vi "test Connect at Local Address.vi"(8 "error in (no error)":errorcluster, 11 "TestCase in":refnum<class "Test TCP Stream Listener Connect.lvclass">) -> (0 "error out":errorcluster, 3 "TestCase out":refnum<class "Test TCP Stream Listener Connect.lvclass">)   [LabVIEW 2020, in "Test TCP Stream Listener Connect.lvclass"]
uses:
  Test TCP Stream Listener Connect.lvclass
  <vilib>/addons/_JKI Toolkits/VI Tester/TestCase.llb/TestCase.lvclass
  Source/Protocols/TCP Strategy/TCP Stream Listener/TCP Stream Listener.lvclass
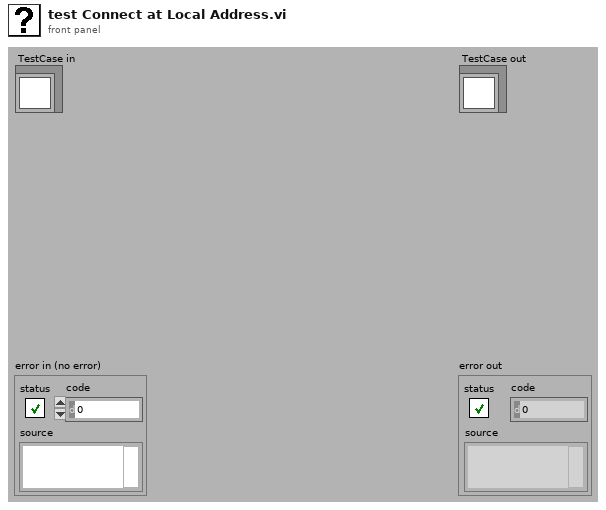
[diagram p1: front panel]
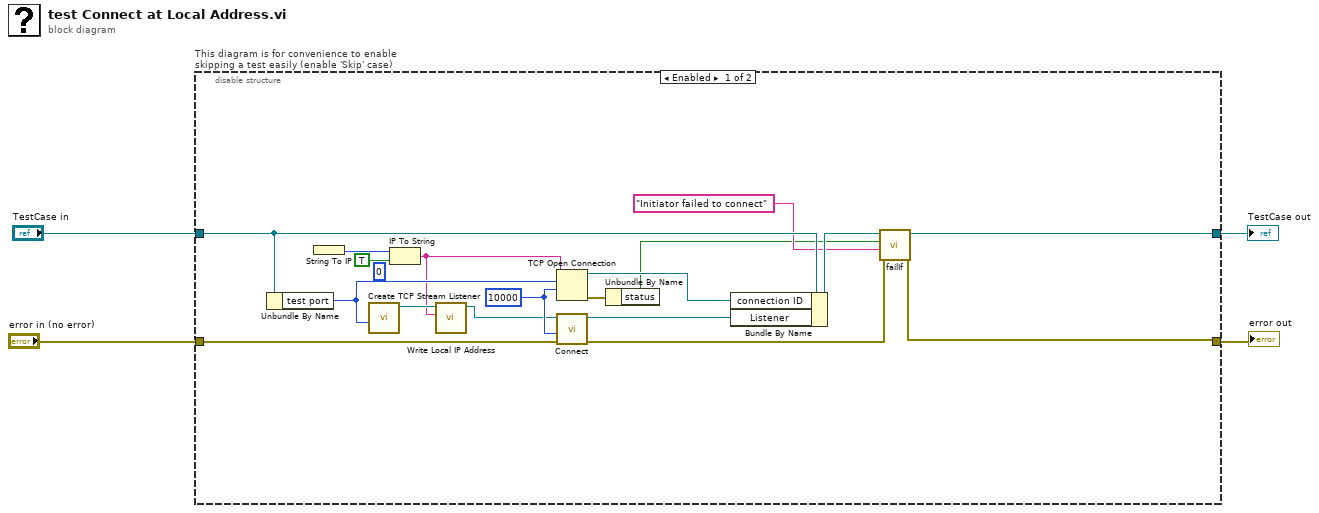
[diagram p0: block diagram]
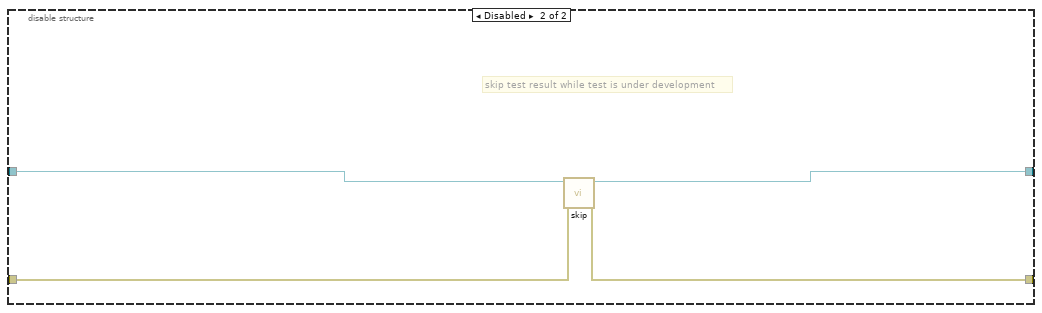
[diagram p2: hidden frame]
diagram:
  n1 = disable-structure "This diagram is for convenience to enable skipping a test easily (enable 'Skip' case)" shown="Enabled" {
    disable-tunnel: "TestCase in" -> [w18 w26]
    disable-tunnel: [w22 w24] -> w1
    disable-tunnel: [w21 w25] -> w3
    disable-tunnel: "error in (no error)" -> [w20 w23]
    frame Enabled {
      (unwired) u32 0 ("net address")
      w13 = 10000 ("timeout")
      n2 = Unbundle By Name(w18) -> ("test port"=w8:u16)
      n3 = String To IP() -> (0:w14:u32)  [unwired: 1 in]
      n4 = call "Create TCP Stream Listener.vi"("Local Port"=w8) -> ("TCP Stream Listener"=w7:refnum<class "TCP Stream Listener.lvclass">)  [unwired: 10 in]
      n5 = IP To String(1:TRUE ("dot notation? (F)"), 2:w14) -> (0:w5:string)
      n6 = call-dynamic "Write Local IP Address.vi"("Local IP"=w5, "TCP Stream Listener in"=w7) -> ("TCP Stream Listener out"=w6:refnum<class "TCP Stream Listener.lvclass">)  [unwired: 9 in]
      n7 = TCP Open Connection(address=w5, remote port or service name=w8, timeout ms (60000)=w13) -> (connection ID=w11:refnum<k5>, error out=w12:errorcluster)  [unwired: 2 in]
      n8 = call-dynamic "Connect.vi"("error in (no error)"=w20, "timeout"=w13, "TCP Stream Listener in"=w6) -> ("error out"=w19:errorcluster, "TCP Stream Listener out"=w9:refnum<class "TCP Stream Listener.lvclass">)  [unwired: 7 in]
      n9 = Unbundle By Name(w12) -> ("status"=w10:bool)
      n10 = Bundle By Name(cluster=w18, "connection ID"=w11, "Listener"=w9) -> (w17:refnum<class "Test TCP Stream Listener Connect.lvclass">)
      n11 = call-dynamic "failIf.vi"("error in (no error)"=w19, "message (\"\")"="Initiator failed to connect" ("message (\"\")"), "fail"=w10, "TestCase in"=w17) -> ("error out"=w21:errorcluster, "TestCase out"=w22:refnum<class "Test TCP Stream Listener Connect.lvclass">)  [unwired: 6 in]
    }
    frame Disabled {
      # "skip test result while test is under development"
      n12 = call <vilib>:"skip.vi"("error in (no error)"=w23, "TestCase in"=w26) -> ("error out"=w25:errorcluster, "TestCase out"=w24:refnum<class "Test TCP Stream Listener Connect.lvclass">)  [unwired: 8 in]
    }
  }
  "error out" <- w3
  "TestCase out" <- w1
